vi "CompareFaces.vi"(7 "tolerance":dbl=0.6, 8 "error in (no error)":errorcluster, 9 "faceEncodingToCheck":refnum<k24>, 10 "knownFaceEncodings":refnum<k24>, 11 "FaceRecognition in":refnum<class "FaceRecognition.lvclass">) -> (0 "error out":errorcluster, 1 "CompareFaces":refnum<k24>, 3 "FaceRecognition out":refnum<class "FaceRecognition.lvclass">)   [LabVIEW 2020, in "FaceRecognitionDotNet.lvlib" / "FaceRecognition.lvclass"]
uses:
  FaceRecognition.lvclass
  dll/FaceRecognitionDotNet.dll
  FaceRecognition.lvclass/FaceRecognition.ctl
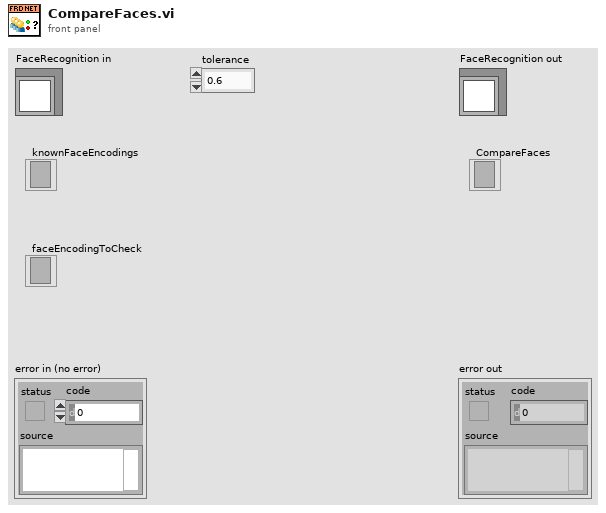
[diagram p1: front panel]
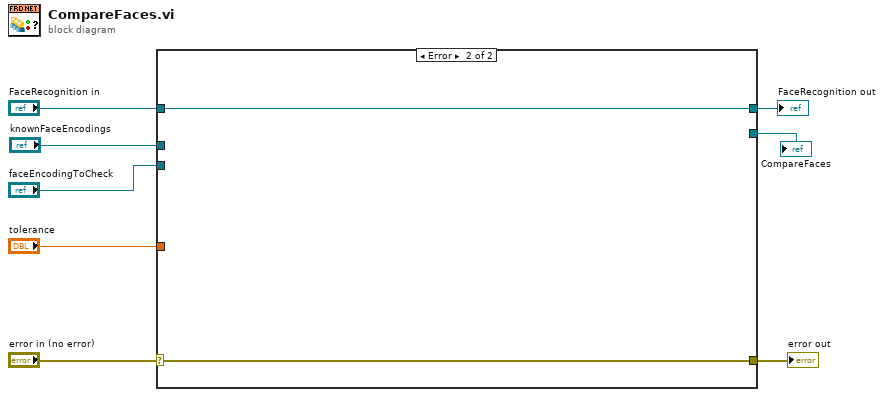
[diagram p0: block diagram]
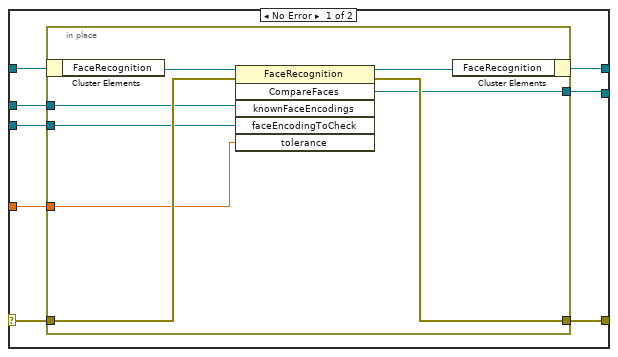
[diagram p2: hidden frame]
diagram:
  n1 = case shown="Error" "error in (no error)" {
    selector: "error in (no error)" -> [w14 w26]
    tunnel: [w13 w26] -> w7
    tunnel: [w15 w25] -> w5
    tunnel: "FaceRecognition in" -> [w16 w25]
    tunnel: [w12 _] -> w1
    tunnel: "faceEncodingToCheck" -> [w11 _]
    tunnel: "tolerance" -> [w10 _]
    tunnel: "knownFaceEncodings" -> [w9 _]
    frame No Error {
      n2 = in-place {
        in-place-border: w14 -> [w22]
        in-place-border: [w21] -> w13
        in-place-border: [w20] -> w12
        in-place-border: w11 -> [w19]
        in-place-border: w10 -> [w18]
        in-place-border: w9 -> [w17]
        n3 = in-place-cluster #1(w16) -> ("FaceRecognition"=w24:refnum<k24>)
        n4 = invoke class="FaceRecognition" method="CompareFaces"(reference=w24, error in=w22, "knownFaceEncodings"=w17, "faceEncodingToCheck"=w19, "tolerance"=w18) -> (reference out=w23:refnum<k24>, error out=w21:errorcluster, "CompareFaces"=w20:refnum<k24>)  [unwired: 1 in, 3 out]
        n5 = in-place-cluster #1("FaceRecognition"=w23) -> (w15:refnum<class "FaceRecognition.lvclass">)
      }
    }
    frame Error {
    }
  }
  "error out" <- w7
  "FaceRecognition out" <- w5
  "CompareFaces" <- w1
